vi "CRC_add.vi"(8 "error in (no error)":errorcluster, 11 "ISO 14443 A UP in":refnum<class "ISO 14443 A UP.lvclass">) -> (0 "error out":errorcluster, 3 "ISO 14443 A UP out":refnum<class "ISO 14443 A UP.lvclass">)   [LabVIEW 2019, in "ISO 14443 A UP.lvclass"]
uses:
  ISO 14443 A UP.lvclass
  TypeDef/Store.ctl
  ISO 14443 A UP.lvclass/ISO 14443 A UP.ctl
  Libraries/CRC/CRC16CITT_A_F.vi
  RFID system.lvclass
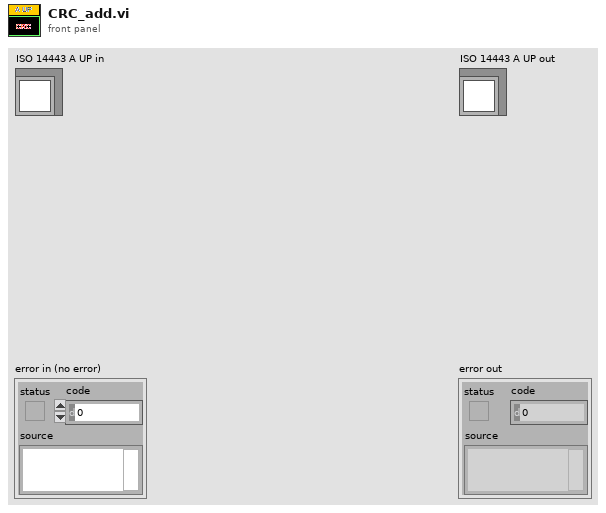
[diagram p1: front panel]
types:
  T1 = typedef "Store.ctl" = enum16{"envelope", "noise", "demSubCar", "CH_frame", "Decode", "demodulate", "in", "out", "sum", "subCarrier", "frame", "command", "encode", "modulate", "encode_UP", "modulate_up", "demod_up", "envelop_up", "sum_up", "out_up", "in_up"}
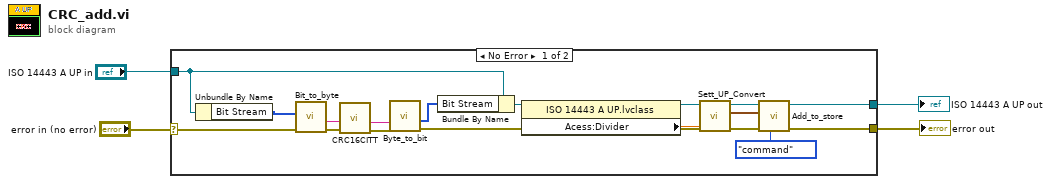
[diagram p0: block diagram]
diagram:
  n1 = case shown="No Error" "error in (no error)" {
    selector: "error in (no error)" -> [w21 w23]
    tunnel: [w12 w23] -> w2
    tunnel: "ISO 14443 A UP in" -> [w20 w24]
    tunnel: [w15 w24] -> w3
    frame No Error {
      n2 = Unbundle By Name(w20) -> ("Bit Stream"=w22:u8[])
      n3 = call "Bit_to_byte.vi"("Error In"=w21, "Array of bit"=w22) -> ("Error Out"=w9:errorcluster, "BYTE"=w10:string)  [unwired: 7 in, 1 out]
      n4 = call-poly "CRC16CITT.vi"("Error In"=w9, "DATA PACKET"=w10) -> ("Error Out"=w8:errorcluster, "DATA PACKET+CRC"=w7:string)  [unwired: 7 in, 1 out]
      n5 = call "Byte_to_bit.vi"("Error In"=w8, "BYTE"=w7) -> ("Error Out"=w13:errorcluster, "Arrray of bit (str)"=w19:u8[])  [unwired: 5 in, 1 out]
      n6 = Bundle By Name(cluster=w20, "Bit Stream"=w19) -> (w18:refnum<class "ISO 14443 A UP.lvclass">)
      n7 = property class="ISO 14443 A UP.lvclass"(reference=w18) -> (reference out=w6:refnum<class "ISO 14443 A UP.lvclass">, "Acess:Divider"=w5:dbl)  [unwired: 1 in, 1 out]
      n8 = call-dynamic "Sett_UP_Convert.vi"("error in (no error)"=w13, "Divider(1)"=w5, "ISO 14443 A UP in"=w6) -> ("error out"=w14:errorcluster, "Waveform"=w17:waveform(dbl), "ISO 14443 A UP out"=w16:refnum<class "ISO 14443 A UP.lvclass">)  [unwired: 6 in]
      n9 = call "Add_to_store.vi"("Store"=Store."command", "error in (no error)"=w14, "Waveform"=w17, "RFID system in"=w16) -> ("error out"=w12:errorcluster, "RFID system out"=w15:refnum<class "ISO 14443 A UP.lvclass">)  [unwired: 6 in]
    }
    frame Error {
    }
  }
  "error out" <- w2
  "ISO 14443 A UP out" <- w3
